vi "Agilent U2000 Series Acquire Measurement Continuously.vi"() -> ()   [LabVIEW 2018]
doc: "This example shows how to acquire power measurements continuously.\n\nNote:\nThis example is not applicable for U2021/2XA."
uses:
  Public/Data/Low Level/Initiate (Continuous).vi
  Agilent U2000 Series.lvlib
panel:
  in  "Stop":bool
  in  "Timeout (10000 ms)":u32=10000
  out "Measurement":dbl
  in  "VISA resource name":refnum<visa-resource-name>
  # "(c) 2014-2015 National Instruments.  ALL RIGHTS RESERVED."
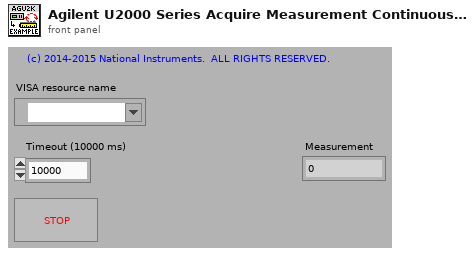
[diagram p1: front panel]
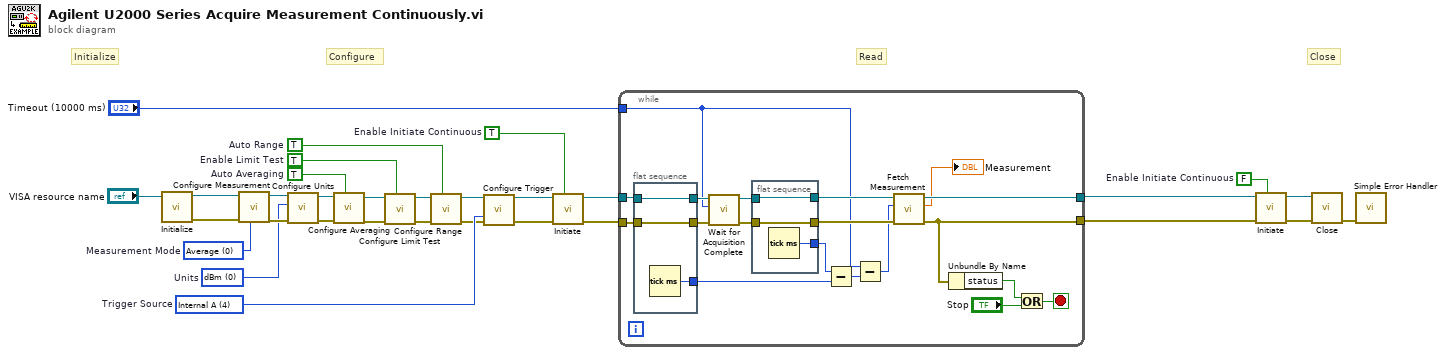
[diagram p0: block diagram]
diagram:
  w5 = FALSE  # Enable Initiate Continuous
  w6 = TRUE  # Enable Initiate Continuous
  w11 = 0 items=["dBm", "Watts"]  # Units
  w24 = 4 items=["Bus", "External", "Hold", "Immediate", "Internal A"]  # Trigger Source
  w25 = 0 items=["Average", "Normal"]  # Measurement Mode
  w17 = TRUE  # Enable Limit Test
  w18 = TRUE  # Auto Averaging
  w16 = TRUE  # Auto Range
  # "Close"
  # "Read"
  # "Configure"
  # "Initialize"
  n1 = call "Initialize.vi"("VISA resource name"="VISA resource name") -> ("error out"=w28:errorcluster, "VISA resource name out"=w29:refnum<visa-resource-name>)  [unwired: 3 in, 6 out]
  n2 = call "Configure Measurement.vi"("Measurement Function (0: Average)"=w25, "error in (no error)"=w28, "VISA resource name"=w29) -> ("error out"=w26:errorcluster, "VISA resource name out"=w27:refnum<visa-resource-name>)  [unwired: 7 in]
  n3 = call "Configure Units.vi"("error in (no error)"=w26, "Units (0: dBm)"=w11, "VISA resource name"=w27) -> ("error out"=w21:errorcluster, "VISA resource name out"=w22:refnum<visa-resource-name>)  [unwired: 1 in, 6 out]
  n4 = call "Configure Averaging.vi"("Enable Averaging (T: Enable)"=w18, "error in (no error)"=w21, "VISA resource name"=w22) -> ("error out"=w19:errorcluster, "VISA resource name out"=w20:refnum<visa-resource-name>)  [unwired: 7 in]
  n5 = call "Configure Limit Test.vi"("Limit Test (T: Enable)"=w17, "error in (no error)"=w19, "VISA resource name"=w20) -> ("error out"=w14:errorcluster, "VISA resource name out"=w15:refnum<visa-resource-name>)  [unwired: 2 in, 5 out]
  n6 = call "Configure Range.vi"("Auto Range (T: Enable)"=w16, "error in (no error)"=w14, "VISA resource name"=w15) -> ("error out"=w13:errorcluster, "VISA resource name out"=w23:refnum<visa-resource-name>)  [unwired: 7 in]
  n7 = call "Configure Trigger.vi"("VISA resource name"=w23, "Trigger Source (3: Immediate)"=w24, "error in (no error)"=w13) -> ("VISA resource name out"=w10:refnum<visa-resource-name>, "error out"=w9:errorcluster)  [unwired: 5 in, 6 out]
  n8 = call-poly "Initiate.vi"("Enable Initiate Continuous (T: Enable)"=w6, "error in (no error)"=w9, "VISA resource name"=w10) -> ("error out"=w7:errorcluster, "VISA resource name out"=w8:refnum<visa-resource-name>)  [unwired: 7 in]
  n9 = while {
    tunnel: w7 -> [w43]
    tunnel: w8 -> [w44]
    tunnel: [w50] -> w4
    tunnel: [w48] -> w3
    tunnel: "Timeout (10000 ms)" -> [w33]
    stop <- w45 stop-if-true
    n10 = flat-sequence {
      tunnel: [w56] -> w42
      tunnel: w44 -> [w56]
      tunnel: [w55] -> w41
      tunnel: w43 -> [w55]
      tunnel: [w54] -> w35
      frame #0 {
        n11 = Tick Count (ms)() -> (millisecond timer value=w54:u32)
      }
    }
    n12 = call "Wait for Acquisition Complete.vi"("error in (no error)"=w41, "Maximum Time (10000 ms)"=w33, "VISA resource name"=w42) -> ("error out"=w39:errorcluster, "VISA resource name out"=w40:refnum<visa-resource-name>)  [unwired: 7 out]
    n13 = flat-sequence {
      tunnel: [w53] -> w38
      tunnel: w40 -> [w53]
      tunnel: [w52] -> w37
      tunnel: w39 -> [w52]
      tunnel: [w51] -> w36
      frame #0 {
        n14 = Tick Count (ms)() -> (millisecond timer value=w51:u32)
      }
    }
    n15 = Subtract(x=w36, y=w35) -> (x-y=w34:u32)
    n16 = Subtract(x=w33, y=w34) -> (x-y=w32:u32)
    n17 = call "Fetch Measurement.vi"("error in (no error)"=w37, "Timeout (10000 ms)"=w32, "VISA resource name"=w38) -> ("error out"=w48:errorcluster, "Measurement"=→"Measurement":dbl, "VISA resource name out"=w50:refnum<visa-resource-name>)  [unwired: 6 in]
    n18 = Unbundle By Name(w48) -> ("status"=w47:bool)
    n19 = Or(x=w47, y="Stop") -> (x .or. y?=w45:bool)
  }
  n20 = call-poly "Initiate.vi"("Enable Initiate Continuous (T: Enable)"=w5, "error in (no error)"=w3, "VISA resource name"=w4) -> ("error out"=w1:errorcluster, "VISA resource name out"=w2:refnum<visa-resource-name>)  [unwired: 7 in]
  n21 = call "Close.vi"("error in (no error)"=w1, "VISA resource name"=w2) -> ("error out"=w30:errorcluster)  [unwired: 9 out]
  n22 = call <vilib>:"Simple Error Handler.vi"("error in (no error)"=w30) -> ()  [unwired: 1 in, 8 out]
